vi "CreateClass.vi"(0 "ClassWriter.lvclass":refnum<class "ClassWriter.lvclass">, 1 "ProjectTreePosition(String or Project Item Ref)":variant, 2 "CreateClassData":T1, 5 "error in (no error)":errorcluster, 6 "KeepLvClassRefOpen(False)":bool, 7 "HeaderToApply (take from VIRef or /use 2D-8bit header, Ignored if not wired)":variant) -> (14 "ClassWriter.lvclass":refnum<class "ClassWriter.lvclass">, 15 "LVClassLibraryRefnum":refnum<vi>, 16 "TemplateVersionUsed":string, 19 "error out":errorcluster)   [LabVIEW 2014, in "ClassWriter.lvclass"]
uses:
  <resource>/Framework/Providers/Open_GDS/ClassProviders/Provider_BaseClassInterface/ClassWriter_class/ClassWriter.lvclass
  <resource>/Framework/Providers/Open_GDS/ClassProviders/Provider_BaseClassInterface/CreateClassData.ctl
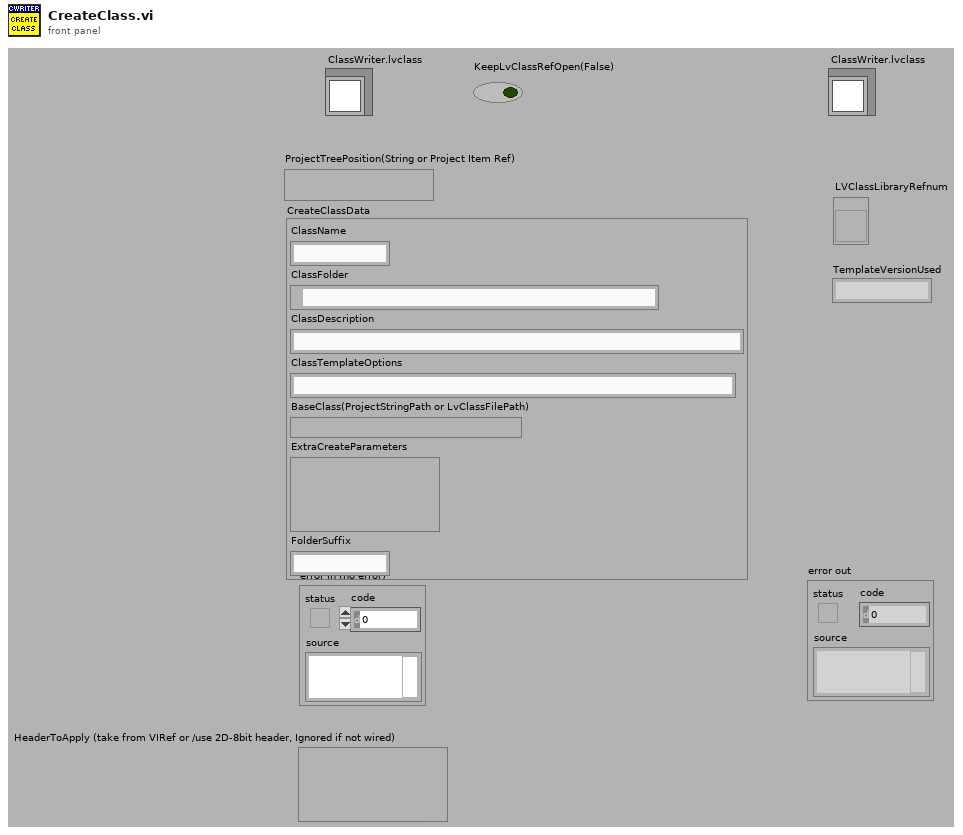
[diagram p1: front panel]
types:
  T1 = typedef "ClassWriter.lvclass/CreateClassData.ctl" = cluster{"ClassName":string, "ClassFolder":path, "ClassDescription":string, "ClassTemplateOptions":string, "BaseClass(ProjectStringPath or LvClassFilePath)":variant, "ExtraCreateParameters":variant, "FolderSuffix":string}
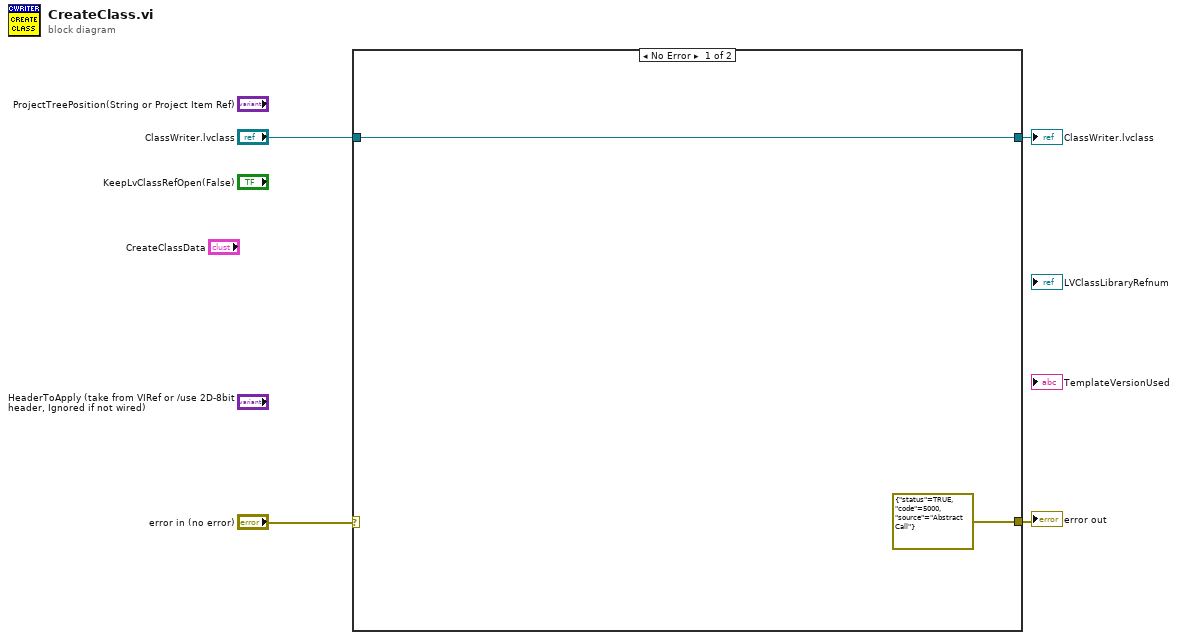
[diagram p0: block diagram]
diagram:
  n1 = case shown="No Error" "error in (no error)" {
    selector: "error in (no error)" -> [_ w7]
    tunnel: "ClassWriter.lvclass" -> [w5 w8]
    tunnel: [errorcluster {"status"=TRUE, "code"=5000, "source"="Abstract Call"} ("error IO") w7] -> w3
    tunnel: [w5 w8] -> w2
    frame No Error {
    }
    frame Error {
    }
  }
  "ClassWriter.lvclass" <- w2
  "error out" <- w3
